vi "Get Waveform.vi"(0 "VISA resource name":refnum<visa-resource-name>, 1 "First Valid Point":i32, 2 "Last Valid Point":i32, 5 "Source (0: Channel 1)":u16(ring) items=["Channel 1", "Channel 2", "Channel 3", "Channel 4", "Memory 1", "Memory 2", "Memory 3", "Memory 4", "Function 1", "Function 2", "Function 3", "Function 4", "Function 5", "Function 6", "Function 7", "Function 8", "Other"], 7 "Command type (0: byte)":u16(ring) items=["Byte", "Word"], 9 "Number Of Data Points (10000)":i32=10000, 11 "error in (no error)":errorcluster, 12 "Timeout (10000 ms)":u32=10000, 13 "Array (0: DAT1)":u16(ring) items=["DAT1", "DAT2"], 14 "Custom Source ID":string) -> (4 "VISA resource name out":refnum<visa-resource-name>, 6 "Waveform Graph":i16[](graph), 15 "error out":errorcluster)   [LabVIEW 2018, in "LeCroy Wave Series.lvlib"]
doc: "Read acquisition waveform from specified source and data block and command format."
uses:
  LeCroy Wave Series.lvlib
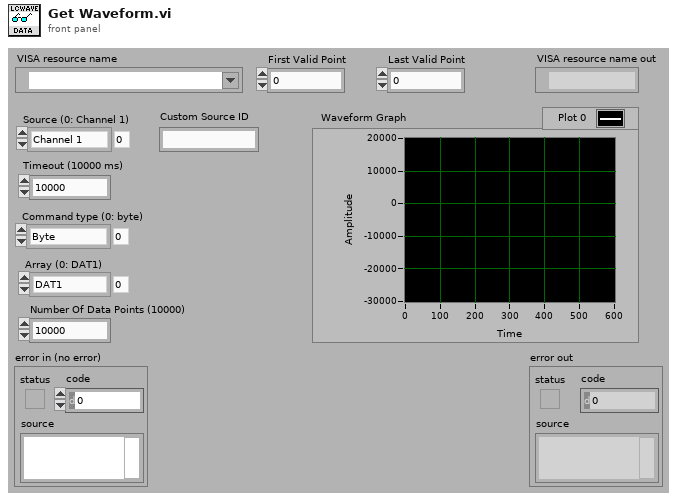
[diagram p1: front panel]
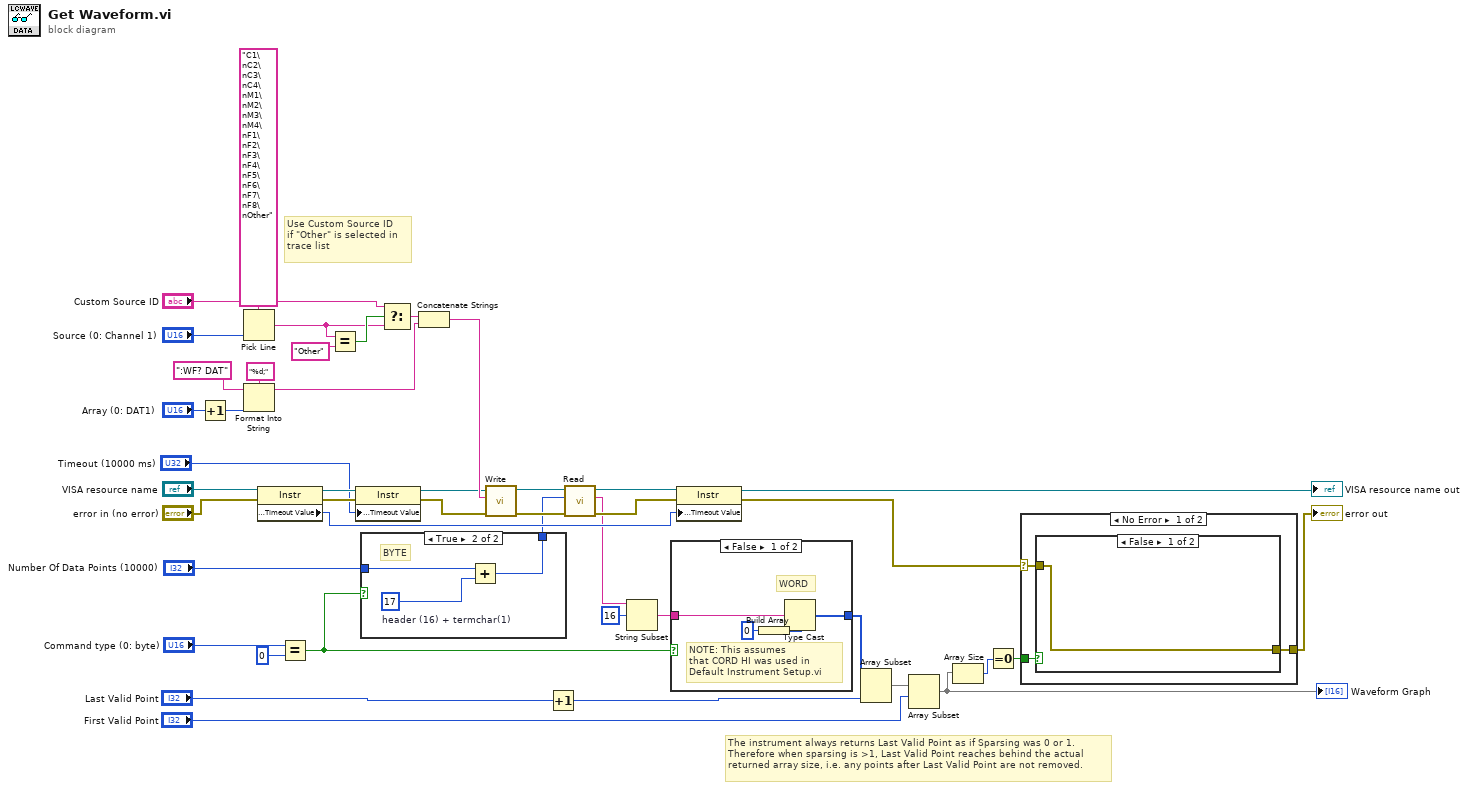
[diagram p0: block diagram]
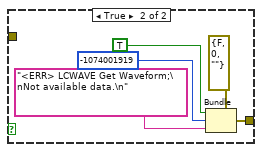
[diagram p2: hidden frame]
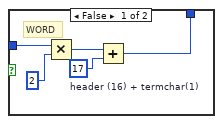
[diagram p4: hidden frame]
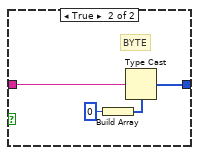
[diagram p5: hidden frame]
diagram:
  # "Use Custom Source ID\nif \"Other\" is selected in \ntrace list"
  # "The instrument always returns Last Valid Point as if Sparsing was 0 or 1.\nTherefore when sparsing is >1, Last Valid Point reaches behind the actual\nreturned array size, i.e. any points after Last Valid Point are not removed."
  n1 = Increment(x="Array (0: DAT1)") -> (x+1=w22:u16)
  n2 = Pick Line(multi-line string="C1\nC2\nC3\nC4\nM1\nM2\nM3\nM4\nF1\nF2\nF3\nF4\nF5\nF6\nF7\nF8\nOther", line index="Source (0: Channel 1)") -> (output string=w3:string)  [unwired: 1 in]
  n3 = Format Into String(format string="%d;", initial string=":WF? DAT" ("write buffer"), w22) -> (resulting string=w35:string)  [unwired: 1 in, 1 out]
  n4 = property on="Property Node" class="Instr"(reference="VISA resource name", error in="error in (no error)") -> (reference out=w32:refnum<visa-resource-name>, error out=w31:errorcluster, "General Settings:Timeout Value"=w25:u32)
  n5 = Equal?(x="Command type (0: byte)", y=u16 0) -> (x = y?=w20:bool)
  n6 = Equal?(x=w3, y="Other" ("x")) -> (x = y?=w6:bool)
  n7 = property on="Property Node" class="Instr"(reference=w32, error in=w31, "General Settings:Timeout Value"="Timeout (10000 ms)") -> (reference out=w30:refnum<visa-resource-name>, error out=w29:errorcluster)
  n8 = case shown="True" w20 {
    tunnel: [w46 w51] -> w21
    tunnel: "Number Of Data Points (10000)" -> [w45 w50]
    frame False {
      w47 = 17  # header (16) + termchar(1)
      # "WORD"
      n9 = Multiply(x=w45, y=2) -> (x*y=w48:i32)
      n10 = Add(x=w48, y=w47) -> (x+y=w46:i32)
    }
    frame True {
      w52 = 17  # header (16) + termchar(1)
      # "BYTE"
      n11 = Add(x=w50, y=w52) -> (x+y=w51:i32)
    }
  }
  n12 = Select(t="Custom Source ID", s=w6, f=w3) -> (s? t:f=w2:string)
  n13 = Concatenate Strings(w2, w35) -> (w44:string)
  n14 = call "Write.vi"("error in (no error)"=w29, "Write Buffer"=w44, "VISA resource name"=w30) -> ("error out"=w42:errorcluster, "VISA resource name out"=w43:refnum<visa-resource-name>)  [unwired: 7 in]
  n15 = Increment(x="Last Valid Point") -> (x+1=w1:i32)
  n16 = call "Read.vi"("error in (no error)"=w42, "Byte Count"=w21, "VISA resource name"=w43) -> ("error out"=w27:errorcluster, "Read Buffer"=w8:string, "VISA resource name out"=w28:refnum<visa-resource-name>)  [unwired: 5 in, 1 out]
  n17 = String Subset(string=w8, offset (0)=16) -> (substring=w7:string)  [unwired: 1 in]
  n18 = case shown="False" w20 {
    tunnel: [w54 w58] -> w15
    tunnel: w7 -> [w53 w57]
    frame False {
      # "NOTE: This assumes\nthat CORD HI was used in Default Instrument Setup.vi"
      # "WORD"
      n19 = Build Array(i16 0) -> (w55:i16[])
      n20 = Type Cast(type=w55, x=w53) -> (*(type *) &x=w54:i16[])
    }
    frame True {
      # "BYTE"
      n21 = Build Array(i8 0) -> (w59:i8[])
      n22 = Type Cast(type=w59, x=w57) -> (*(type *) &x=w58:i8[])
    }
  }
  n23 = property on="Property Node" class="Instr"(reference=w28, error in=w27, "General Settings:Timeout Value"=w25) -> (reference out=→"VISA resource name out":refnum<visa-resource-name>, error out=w11:errorcluster)
  n24 = Array Subset(array=w15, length=w1) -> (w18:i16[])  [unwired: 1 in]
  n25 = Array Subset(array=w18, index="First Valid Point") -> (w13:i16[])  [unwired: 1 in]
  "Waveform Graph" <- w13
  n26 = Array Size(array=w13) -> (size(s)=w12:i32)
  n27 = Equal To 0?(x=w12) -> (x = 0?=w10:bool)
  n28 = case shown="No Error" w11 {
    selector: w11 -> [w61 w70]
    tunnel: [w63 w70] -> w14
    tunnel: w10 -> [w62 _]
    frame No Error {
      n29 = case shown="False" w62 {
        tunnel: [w64 w65] -> w63
        tunnel: w61 -> [w64 _]
        frame False {
        }
        frame True {
          n30 = Bundle(cluster=errorcluster {"status"=FALSE, "code"=0, "source"=""} ("error out"), "status"=TRUE, "code"=-1074001919 ("Code"), "source"="<ERR> LCWAVE Get Waveform;\nNot available data.\n" ("Source")) -> (w65:errorcluster)
        }
      }
    }
    frame Error {
    }
  }
  "error out" <- w14
